vi "Write StreamTX filename.vi"(8 "error in (no error)":errorcluster, 10 "StreamTX filename":string, 11 "Stream in":refnum<class "Stream.lvclass">) -> (0 "error out":errorcluster, 3 "Stream out":refnum<class "Stream.lvclass">)   [LabVIEW 2018, in "Stream.lvclass"]
uses:
  Stream.lvclass
  Stream.lvclass/Stream.ctl
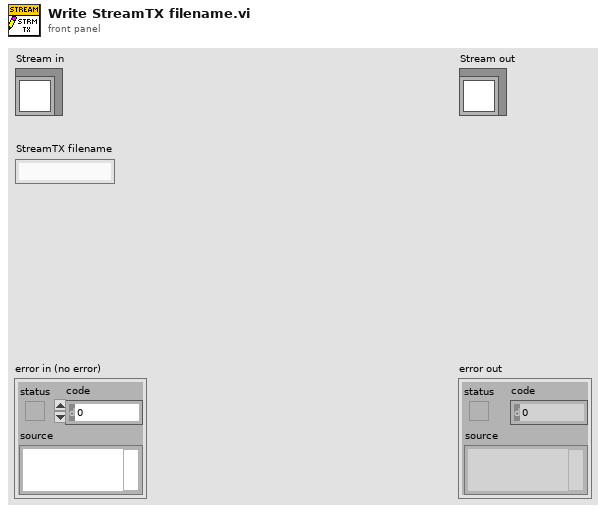
[diagram p1: front panel]
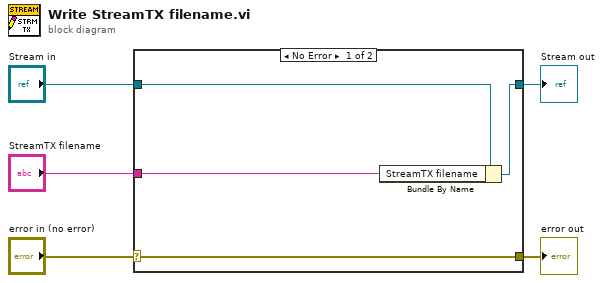
[diagram p0: block diagram]
diagram:
  n1 = case shown="No Error" "error in (no error)" {
    selector: "error in (no error)" -> [w9 w10]
    tunnel: [w9 w10] -> w4
    tunnel: [w7 w11] -> w2
    tunnel: "Stream in" -> [w8 w11]
    tunnel: "StreamTX filename" -> [w6 _]
    frame No Error {
      n2 = Bundle By Name(cluster=w8, "StreamTX filename"=w6) -> (w7:refnum<class "Stream.lvclass">)
    }
    frame Error {
    }
  }
  "error out" <- w4
  "Stream out" <- w2
